vi "VI Server Setup.vi"(9 "This VI":refnum<vi>, 10 "This Application":refnum<vi>, 11 "Base jettl in":refnum<class "Base jettl.lvclass">) -> (3 "Base jettl out":refnum<class "Base jettl.lvclass">)   [LabVIEW 2021, in "jettl.lvlib" / "Base jettl.lvclass"]
uses:
  Base jettl.lvclass
  Base jettl.lvclass/Base jettl.ctl
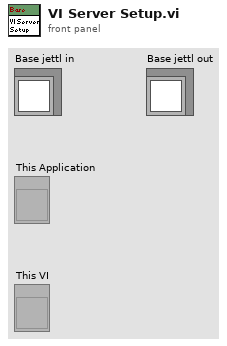
[diagram p1: front panel]
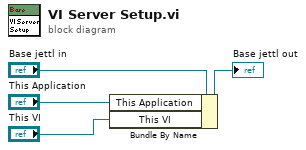
[diagram p0: block diagram]
diagram:
  n1 = Bundle By Name(cluster="Base jettl in", "This Application"="This Application", "This VI"="This VI") -> (→"Base jettl out":refnum<class "Base jettl.lvclass">)
